vi "Get All Objects.vi"(8 "error in (no error)":errorcluster, 11 "Objects in":refnum<class "Objects.lvclass">) -> (0 "error out":errorcluster, 1 "Objects":refnum<class "Object.lvclass">[](array[class]), 3 "Objects out":refnum<class "Objects.lvclass">)   [LabVIEW 2019, in "HierDAL Library.lvlib" / "Database.lvlib" / "Repositories.lvlib" / "Objects.lvclass"]
uses:
  Objects.lvclass
  Models Library/Object Class/Object.lvclass
  Objects.lvclass/Objects.ctl
  46314e7c-a004-450c-aec5-182bd9d357fe.vi
  Database Manager Class/Database Manager.lvclass
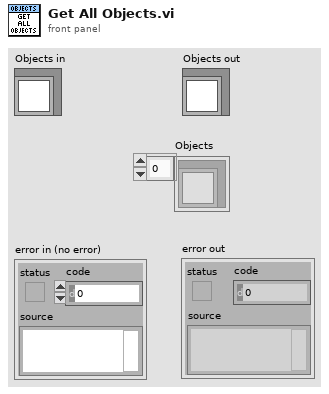
[diagram p1: front panel]
types:
  T1 = typedef "HierDAL Library.lvlib/Common.lvlib/Datatype.ctl" = enum16{"Unknown", "Group", "Dataset"}
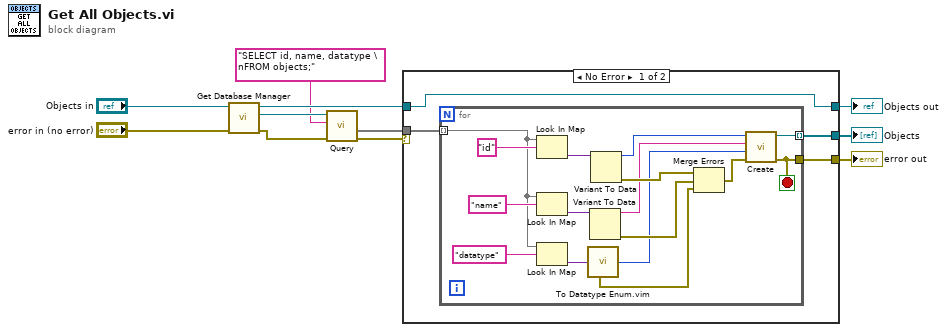
[diagram p0: block diagram]
diagram:
  n1 = call "Get Database Manager.vi"("error in (no error)"="error in (no error)", "Objects in"="Objects in") -> ("error out"=w10:errorcluster, "Database Manager"=w9:refnum<class "Database Manager.lvclass">, "Objects out"=w11:refnum<class "Objects.lvclass">)  [unwired: 7 in]
  n2 = call-dynamic "Query.vi"("error in (no error)"=w10, "Query"="SELECT id, name, datatype \nFROM objects;", "Database Manager in"=w9) -> ("error out"=w3:errorcluster, "Rows"=w5:map{string, variant}[])  [unwired: 6 in, 1 out]
  n3 = case shown="No Error" w3 {
    selector: w3 -> [_ w32]
    tunnel: [w15 _] -> w1
    tunnel: w5 -> [w12 _]
    tunnel: [w14 w32] -> w4
    tunnel: w11 -> [w13 w33]
    tunnel: [w13 w33] -> w2
    frame No Error {
      n4 = for {
        tunnel: [w31] -> w15 mode=indexing
        tunnel: [w19] -> w14
        tunnel: w12 -> [w20] mode=indexing
        stop <- w19 stop-if-true
        n5 = Look In Map(map=w20, key="id") -> (value=w27:variant)  [unwired: 1 in, 1 out]
        n6 = Look In Map(map=w20, key="name") -> (value=w26:variant)  [unwired: 1 in, 1 out]
        n7 = Look In Map(map=w20, key="datatype") -> (value=w22:variant)  [unwired: 1 in, 1 out]
        n8 = call "To Datatype Enum.vim"("Value"=w22) -> ("error out"=w21:errorcluster, "Datatype"=w16:T1)  [unwired: 5 in]
        n9 = Variant To Data(Variant=w26) -> (data=w17:string, error out=w24:errorcluster)  [unwired: 2 in]
        n10 = Variant To Data(Variant=w27) -> (data=w18:i32, error out=w25:errorcluster)  [unwired: 2 in]
        n11 = Merge Errors(w25, w24, w21) -> (w23:errorcluster)
        n12 = call "Create.vi"("error in (no error)"=w23, "Datatype"=w16, "Name"=w17, "ID"=w18) -> ("error out"=w19:errorcluster, "Object out"=w31:refnum<class "Object.lvclass">)  [unwired: 6 in]
      }
    }
    frame Error {
    }
  }
  "error out" <- w4
  "Objects out" <- w2
  "Objects" <- w1
